vi "Lookup Groups.vi"(8 "error in (no error)":errorcluster, 11 "DAQmxAI in":refnum<class "DAQmxAI.lvclass">) -> (0 "error out":errorcluster, 2 "Channels":refnum<class "Group Config.lvclass">, 3 "DAQmxAI out":refnum<class "DAQmxAI.lvclass">, 4 "Commands":refnum<class "Group Config.lvclass">)   [LabVIEW 2023, in "VolatusDAQ.lvlib" / "DAQmxAI.lvclass"]
uses:
  DAQmxAI.lvclass
  DAQmxAI.lvclass/DAQmxAI.ctl
  Volatus/Module/Module.lvclass
  VolatusConfig/Task/Task Config.lvclass
  VolatusConfig/VolatusConfigElement/VolatusConfigElement.lvclass
  C:/dev/volatus/mts-volatus-super/libs/lv-volatus/Volatus/Module/Module.lvclass
  C:/dev/volatus/mts-volatus-super/libs/lv-volatus/VolatusDAQ/DAQmxAI/DAQmxAI.lvclass
  VolatusConfig/Group/Group Config.lvclass
  C:/dev/volatus/mts-volatus-super/libs/lv-volatus/VolatusConfig/VolatusConfigElement/VolatusConfigElement.lvclass
  C:/dev/volatus/mts-volatus-super/libs/lv-volatus/VolatusConfig/Group/Group Config.lvclass
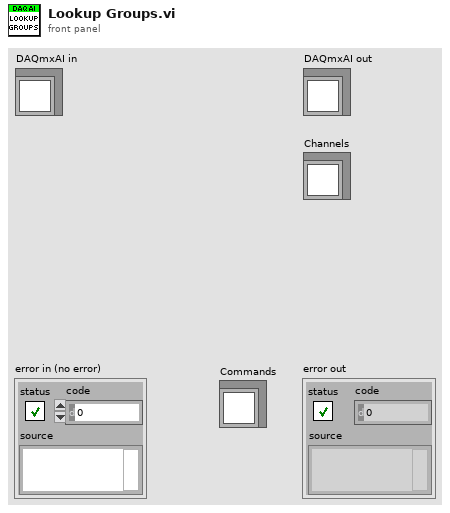
[diagram p1: front panel]
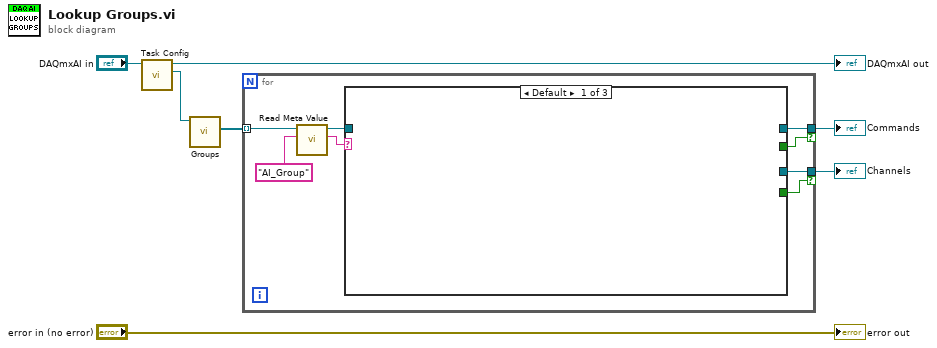
[diagram p0: block diagram]
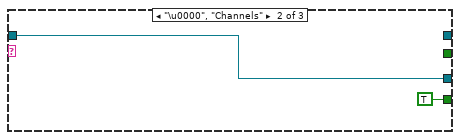
[diagram p2: hidden frame]
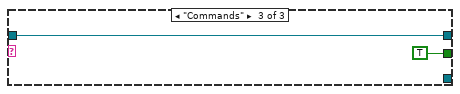
[diagram p3: hidden frame]
diagram:
  n1 = call "Task Config.vi"("Module in"="DAQmxAI in") -> ("Task Config"=w4:refnum<class "Task Config.lvclass">, "Module out"=→"DAQmxAI out":refnum<class "DAQmxAI.lvclass">)  [unwired: 8 in, 1 out]
  n2 = call "Groups.vi"("Task in"=w4) -> ("Groups"=w3:refnum<class "Group Config.lvclass">[])  [unwired: 8 in, 2 out]
  n3 = for {
    tunnel: w3 -> [w15] mode=indexing
    tunnel: [w11] -> w2 if=w10
    tunnel: [w9] -> w1 if=w8
    n4 = call "Read Meta Value.vi"("Meta Name"="AI_Group", "VolatusConfigElement in"=w15) -> ("Meta Value"=w13:string, "VolatusConfigElement out"=w12:refnum<class "Group Config.lvclass">)  [unwired: 7 in, 1 out]
    n5 = case shown="Default" w13 {
      tunnel: w12 -> [_ w17 w19]
      tunnel: [_ _ w19] -> w11
      tunnel: [_ _ TRUE] -> w10
      tunnel: [_ w17 _] -> w9
      tunnel: [_ TRUE _] -> w8
      frame Default {
      }
      frame "\u0000", "Channels" {
      }
      frame "Commands" {
      }
    }
  }
  "Commands" <- w2
  "Channels" <- w1
  "error out" <- "error in (no error)"
